vi "AgB29xx_LabVIEW_StaircaseSweep.vi"() -> ()   [LabVIEW 2009]
panel:
  out "InstrumentFirmwareRevision":string
  out "Simulate":bool
  out "SerialNumber":string
  out "Identifier":string
  out "Revision":string
  out "Vendor":string
  out "Description":string
  out "InstrumentModel":string
  in  "OptionString":string="QueryInstrStatus=true, Simulate=true, DriverSetup= Model=, Trace=false"
  in  "Reset":bool=TRUE
  in  "IdQuery":bool=TRUE
  in  "ResourceName":string="GPIB0::23::INSTR"
  out "Items":string
  out "iNumberOfChannels":i32=2
  out "data":dbl[](array[numeric])
  in  "AgB29xxLib.IAgB29xx2":refnum<k7>
  # "Staircase Sweep"
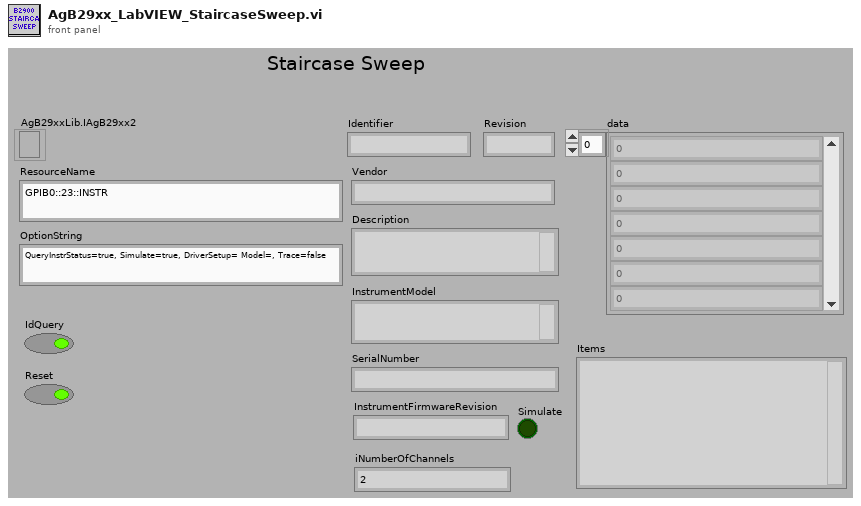
[diagram p1: front panel]
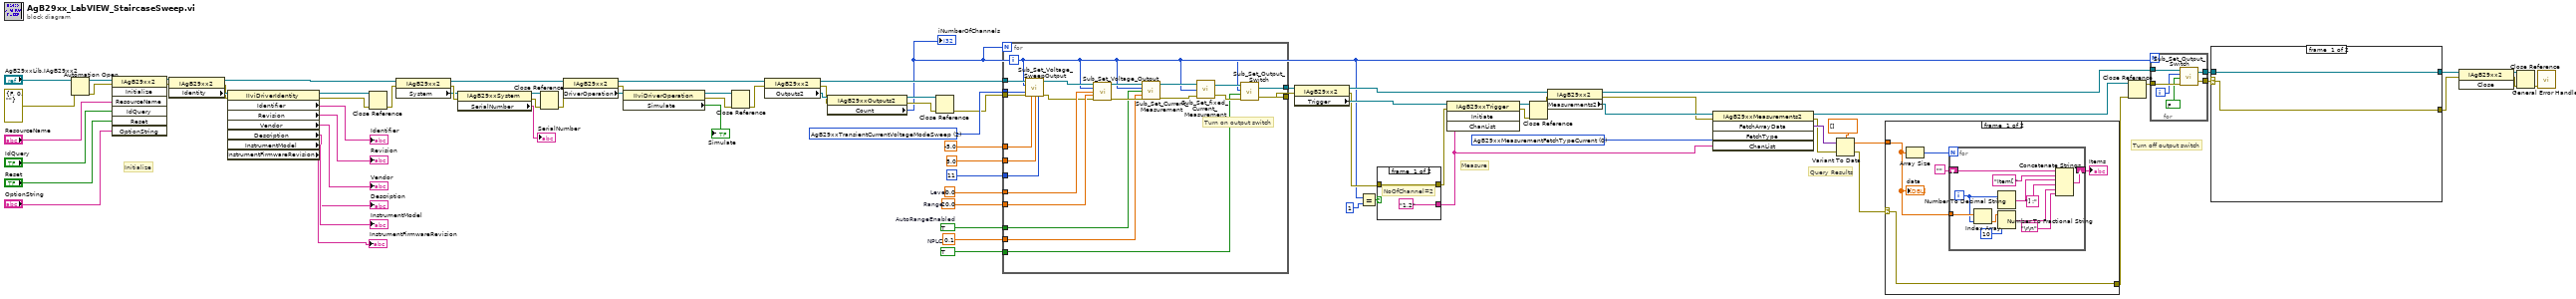
[diagram p0: block diagram]
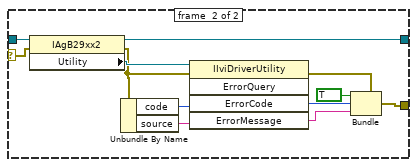
[diagram p2: hidden frame]
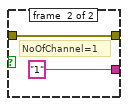
[diagram p4: hidden frame]
diagram:
  w58 = 2 items=["AgB29xxTransientCurrentVoltageModeFixed", "AgB29xxTransientCurrentVoltageModeList", "AgB29xxTransientCurrentVoltageModeSweep"] ("Mode")
  w60 = TRUE  # AutoRangeEnabled
  w61 = 0.1  # NPLC
  w62 = 20.0  # Range
  w63 = 0.0  # Level
  w77 = 0 items=["AgB29xxMeasurementFetchTypeCurrent", "AgB29xxMeasurementFetchTypeResistance", "AgB29xxMeasurementFetchTypeSource", "AgB29xxMeasurementFetchTypeStatus", "AgB29xxMeasurementFetchTypeTime", "AgB29xxMeasurementFetchTypeVoltage", "AgB29xxMeasurementFetchTypeAll"] ("FetchType")
  # "Turn off output switch"
  # "Query Results"
  # "Measure"
  # "Initialize"
  n1 = Automation Open(error in (no error)=errorcluster {"status"=FALSE, "code"=0, "source"=""}, Automation Refnum="AgB29xxLib.IAgB29xx2") -> (Automation Refnum=w81:refnum<k7>, error out=w82:errorcluster)  [unwired: 2 in]
  n2 = invoke class="IAgB29xx2" method="Initialize"(reference=w81, error in=w82, "ResourceName"="ResourceName", "IdQuery"="IdQuery", "Reset"="Reset", "OptionString"="OptionString") -> (reference out=w24:refnum<k7>, error out=w23:errorcluster)  [unwired: 1 in, 5 out]
  n3 = property class="IAgB29xx2"(reference=w24, error in=w23) -> (reference out=w49:refnum<k7>, error out=w52:errorcluster, "Identity"=w53:refnum<k7>)
  n4 = property class="IIviDriverIdentity"(reference=w53, error in=w52) -> (reference out=w48:refnum<k7>, error out=w47:errorcluster, "Identifier"=→"Identifier":string, "Revision"=→"Revision":string, "Vendor"=→"Vendor":string, "Description"=→"Description":string, "InstrumentModel"=→"InstrumentModel":string, "InstrumentFirmwareRevision"=→"InstrumentFirmwareRevision":string)
  n5 = Close Reference(reference=w48, error in (no error)=w47) -> (error out=w46:errorcluster)
  n6 = property class="IAgB29xx2"(reference=w49, error in=w46) -> (reference out=w43:refnum<k7>, error out=w51:errorcluster, "System"=w50:refnum<k7>)
  n7 = property class="IAgB29xxSystem"(reference=w50, error in=w51) -> (reference out=w41:refnum<k7>, error out=w42:errorcluster, "SerialNumber"=→"SerialNumber":string)
  n8 = Close Reference(reference=w41, error in (no error)=w42) -> (error out=w40:errorcluster)
  n9 = property class="IAgB29xx2"(reference=w43, error in=w40) -> (reference out=w26:refnum<k7>, error out=w44:errorcluster, "DriverOperation"=w45:refnum<k7>)
  n10 = property class="IIviDriverOperation"(reference=w45, error in=w44) -> (reference out=w39:refnum<k7>, error out=w38:errorcluster, "Simulate"=→"Simulate":bool)
  n11 = Close Reference(reference=w39, error in (no error)=w38) -> (error out=w25:errorcluster)
  n12 = property class="IAgB29xx2"(reference=w26, error in=w25) -> (reference out=w22:refnum<k7>, error out=w28:errorcluster, "Outputs2"=w30:refnum<k7>)
  n13 = property class="IAgB29xxOutputs2"(reference=w30, error in=w28) -> (reference out=w29:refnum<k7>, error out=w27:errorcluster, "Count"=w3:i32)
  "iNumberOfChannels" <- w3
  n14 = Close Reference(reference=w29, error in (no error)=w27) -> (error out=w21:errorcluster)
  n15 = for {
    N: w3 -> [_]
    tunnel: [w102] -> w70
    tunnel: [w101] -> w68
    tunnel: w63 -> [w100]
    tunnel: w62 -> [w99]
    tunnel: w61 -> [w97]
    tunnel: w60 -> [w96]
    tunnel: TRUE ("Enabled? (False)") -> [w92]
    tunnel: w58 -> [w91]
    tunnel: -5.0 ("Start") -> [w90]
    tunnel: 5.0 ("Stop") -> [w89]
    tunnel: u32 11 ("Sweep Points") -> [w88]
    tunnel: w22 -> [w86]
    tunnel: w21 -> [w85]
    i -> [w84]
    # "Turn on output switch"
    n16 = call "Sub_Set_Voltage_SweepOutput.vi"("AgB29xxLib.IAgB29xx2"=w86, "i"=w84, "Mode"=w91, "error in (no error)"=w85, "Start"=w90, "Stop"=w89, "Sweep Points"=w88) -> ("AgB29xxLib.IAgB29xx2 2"=w105:refnum<k7>, "error out"=w98:errorcluster)  [unwired: 7 in]
    n17 = call "Sub_Set_Voltage_Output.vi"("AgB29xxLib.IAgB29xx2"=w105, "i"=w84, "Level"=w100, "Range"=w99, "error in"=w98) -> ("AgB29xxLib.IAgB29xx2 2"=w104:refnum<k7>, "error out"=w103:errorcluster)  [unwired: 9 in]
    n18 = call "Sub_Set_Current_Measurement.vi"("AgB29xxLib.IAgB29xx2"=w104, "i"=w84, "AutoRangeEnabled"=w96, "NPLC"=w97, "error in"=w103) -> ("AgB29xxLib.IAgB29xx2 2"=w87:refnum<k7>, "error out"=w95:errorcluster)  [unwired: 9 in]
    n19 = call "Sub_Set_fixed_Current_Measurement.vi"("error in"=w95, "i"=w84, "AgB29xxLib.IAgB29xx2"=w87) -> ("error out"=w94:errorcluster, "AgB29xxLib.IAgB29xx2 2"=w93:refnum<k7>)
    n20 = call "Sub_Set_Output_Switch.vi"("error in"=w94, "Enabled? (False)"=w92, "i"=w84, "AgB29xxLib.IAgB29xx2"=w93) -> ("error out"=w101:errorcluster, "AgB29xxLib.IAgB29xx2 2"=w102:refnum<k7>)
  }
  n21 = property class="IAgB29xx2"(reference=w70, error in=w68) -> (reference out=w64:refnum<k7>, error out=w17:errorcluster, "Trigger"=w69:refnum<k7>)
  n22 = Equal?(x=w3, y=1 ("iStart")) -> (x = y?=w19:bool)
  n23 = case shown="False" w19 {
    tunnel: ["1,2" "1"] -> w15
    tunnel: w17 -> [w106 w108]
    tunnel: [w106 w108] -> w16
    frame #0 {
      # "NoOfChannel=2"
    }
    frame #1 {
      # "NoOfChannel=1"
    }
  }
  n24 = invoke class="IAgB29xxTrigger" method="Initiate"(reference=w69, error in=w16, "ChanList"=w15) -> (reference out=w67:refnum<k7>, error out=w66:errorcluster)  [unwired: 1 in, 2 out]
  n25 = Close Reference(reference=w67, error in (no error)=w66) -> (error out=w65:errorcluster)
  n26 = property class="IAgB29xx2"(reference=w64, error in=w65) -> (reference out=w2:refnum<k7>, error out=w74:errorcluster, "Measurements2"=w78:refnum<k7>)
  n27 = invoke class="IAgB29xxMeasurements2" method="FetchArrayData"(reference=w78, error in=w74, "FetchType"=w77, "ChanList"=w15) -> (reference out=w1:refnum<k7>, error out=w54:errorcluster, "FetchArrayData"=w75:variant)  [unwired: 1 in, 2 out]
  n28 = Variant To Data(error in=w54, Variant=w75, type=dbl[] []) -> (error out=w4:errorcluster, data=w5:dbl[])
  n29 = case shown="No Error" w4 {
    selector: w4 -> [w113 w126]
    tunnel: w5 -> [w111 _]
    tunnel: [w113 w126] -> w10
    frame #0 {
      n30 = Array Size(array=w111) -> (size(s)=w112:i32)
      n31 = for {
        N: w112 -> [_]
        tunnel: w111 -> [w121]
        shift-right: [w118] -> w110
        shift-left: "" -> [w117]
        i -> [w116]
        n32 = Index Array(array=w121, index=w116) -> (element=w120:dbl)
        n33 = Number To Decimal String(number=w116) -> (decimal integer string=w124:string)  [unwired: 1 in]
        n34 = Number To Fractional String(number=w120, precision (6)=i16 10) -> (F-format string=w122:string)  [unwired: 2 in]
        n35 = Concatenate Strings(w117, "Item[ " ("string"), w124, "] :" ("string"), w122, "\r\n") -> (w118:string)
      }
      "Items" <- w110
      "data" <- w111
    }
    frame #1 {
    }
  }
  n36 = Close Reference(reference=w1, error in (no error)=w10) -> (error out=w12:errorcluster)
  n37 = for {
    N: w3 -> [_]
    tunnel: w2 -> [w132]
    tunnel: w12 -> [w131]
    tunnel: [w129] -> w9
    tunnel: [w128] -> w8
    i -> [w127]
    n38 = call "Sub_Set_Output_Switch.vi"("error in"=w131, "Enabled? (False)"=FALSE ("AutoRangeEnabled"), "i"=w127, "AgB29xxLib.IAgB29xx2"=w132) -> ("error out"=w129:errorcluster, "AgB29xxLib.IAgB29xx2 2"=w128:refnum<k7>)
  }
  n39 = case shown="Error" w9 {
    selector: w9 -> [w133 w145]
    tunnel: [w133 w135] -> w6
    tunnel: w8 -> [w134 w146]
    tunnel: [w134 w143] -> w7
    frame #0 {
    }
    frame #1 {
      n40 = property class="IAgB29xx2"(reference=w146, error in=w145) -> (reference out=w143:refnum<k7>, error out=w140:errorcluster, "Utility"=w144:refnum<k7>)
      n41 = Unbundle By Name(w140) -> ("code"=w142:i32, "source"=w141:string)
      n42 = invoke class="IIviDriverUtility" method="ErrorQuery"(reference=w144, error in=w140, "ErrorCode"=w142, "ErrorMessage"=w141) -> (error out=w136:errorcluster, "ErrorCode"=w139:i32, "ErrorMessage"=w138:string)  [unwired: 1 in, 2 out]
      n43 = Bundle(cluster=w136, "status"=TRUE, "code"=w139, "source"=w138) -> (w135:errorcluster)
    }
  }
  n44 = invoke class="IAgB29xx2" method="Close"(reference=w7, error in=w6) -> (reference out=w14:refnum<k7>, error out=w13:errorcluster)  [unwired: 1 in, 1 out]
  n45 = Close Reference(reference=w14, error in (no error)=w13) -> (error out=w11:errorcluster)
  n46 = call <vilib>:"General Error Handler.vi"("error in (no error)"=w11) -> ()  [unwired: 10 in, 5 out]
